vi "DrawPoints.vi"(2 "error in (no error)":errorcluster, 3 "Points":cluster{"Edge Info":T2, "Boolean":bool}[](array[cluster]) {"Edge Info"."Distance (Real-World)" format="%.2f"; "Edge Info"."Location (Real-World)"."Y" format="%.2g"; "Edge Info"."Location (Real-World)"."X" format="%.2f"; "Edge Info"."Noise" format="%.2f"; "Edge Info"."Location (Pixel)"."Y" format="%.2g"; "Edge Info"."Location (Pixel)"."X" format="%.2f"; "Edge Info"."Strength" format="%.2f"; "Edge Info"."Distance (Pixel)" format="%.2f"}, 4 "Image in":T1) -> (0 "error out":errorcluster, 1 "Image Out":T1)   [LabVIEW 2015]
uses:
  <vilib>/vision/Measure.llb/Edge New.ctl
  <vilib>/vision/Image Controls.llb/IMAQ Image.ctl
panel:
  out "Image":T1(plugin-control)
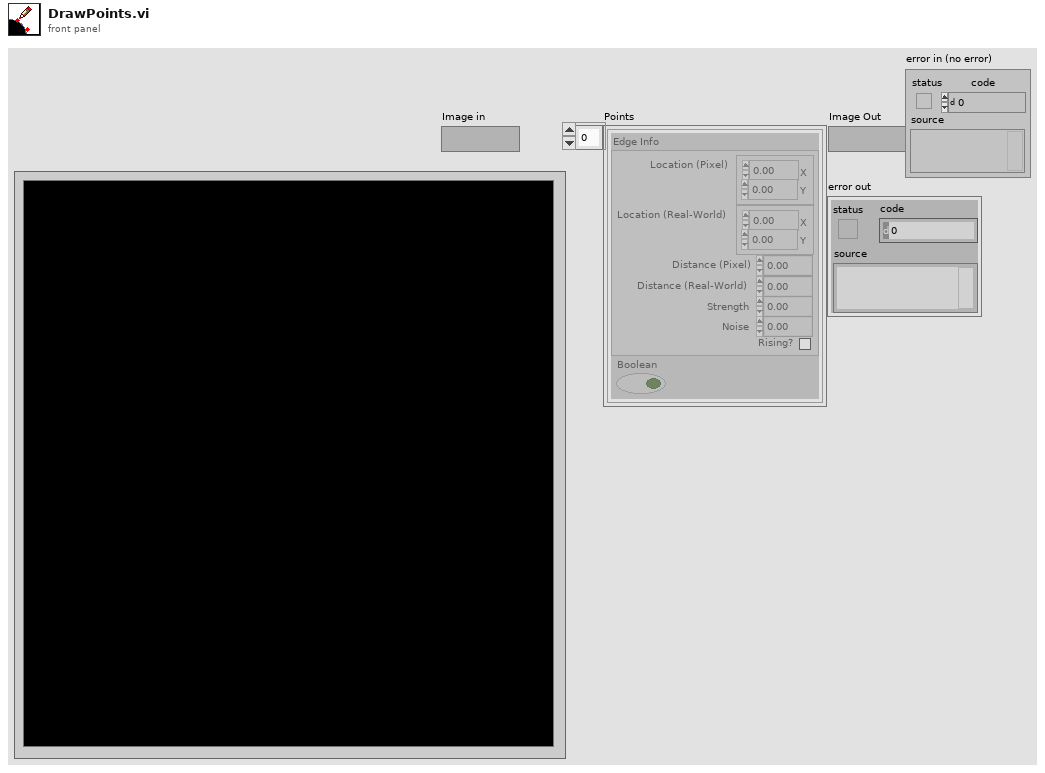
[diagram p1: front panel]
types:
  T1 = typedef "IMAQ Image.ctl" = refnum<image>
  T2 = typedef "Edge New.ctl" = cluster{"Location (Pixel)":cluster{"X":sgl, "Y":sgl}, "Location (Real-World)":cluster{"X":sgl, "Y":sgl}, "Distance (Pixel)":dbl, "Distance (Real-World)":dbl, "Strength":dbl, "Noise":dbl, "Rising?":bool}
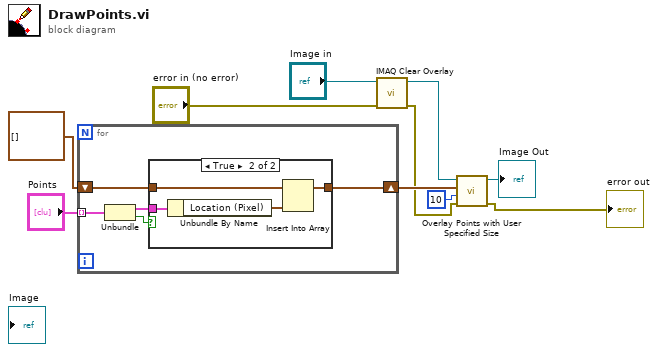
[diagram p0: block diagram]
diagram:
  n1 = for {
    tunnel: "Points" -> [w14] mode=indexing
    shift-right: [w15] -> w9
    shift-left: cluster{"X":sgl, "Y":sgl}[] [] ("array") -> [w11]
    n2 = Unbundle(w14) -> ("Edge Info"=w13:T2, "Boolean"=w12:bool)
    n3 = case shown="True" w12 {
      tunnel: [w16 w18] -> w15
      tunnel: w13 -> [_ w20]
      tunnel: w11 -> [w16 w17]
      frame False {
      }
      frame True {
        n4 = Unbundle By Name(w20) -> ("Location (Pixel)"=w19:cluster{"X":sgl, "Y":sgl})
        n5 = Insert Into Array(array=w17, new element=w19) -> (w18:cluster{"X":sgl, "Y":sgl}[])  [unwired: 1 in]
      }
    }
  }
  n6 = call "IMAQ Clear Overlay"("error in (no error)"="error in (no error)", "Image"="Image in") -> ("error out"=w2:errorcluster, "Image Out"=w10:T1)  [unwired: 8 in]
  n7 = call "Overlay Points with User Specified Size.vi"("error in"=w2, "Point Diameter (5)"=u32 10, "Points"=w9, "Image In"=w10) -> ("error out"=→"error out":errorcluster, "Image Out"=→"Image Out":T1)  [unwired: 6 in]
